vi "generateArrays.vi"(0 "dimension size":i32) -> (8 "errorsWindow1":dbl[](array[numeric]), 10 "pckTotalTrack1":dbl[](array[numeric]), 12 "state1":dbl[](array[numeric]), 14 "errorsWindow2":dbl[](array[numeric]), 15 "pckTotalTrack2":dbl[](array[numeric]), 16 "state2":dbl[](array[numeric]), 17 "errorsWindow3":dbl[](array[numeric]), 18 "pckTotalTrack3":dbl[](array[numeric]), 19 "state3":dbl[](array[numeric]))   [LabVIEW 2010]
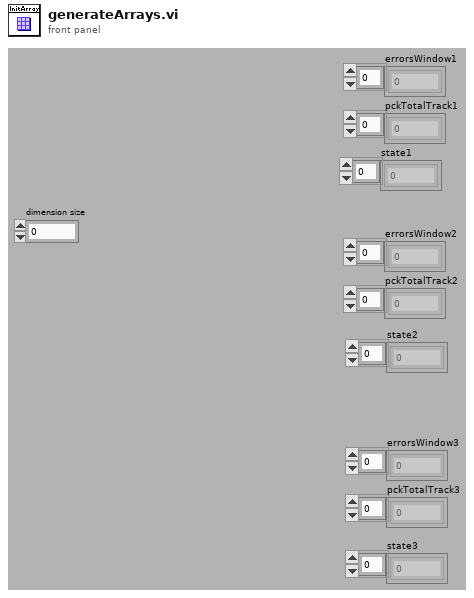
[diagram p1: front panel]
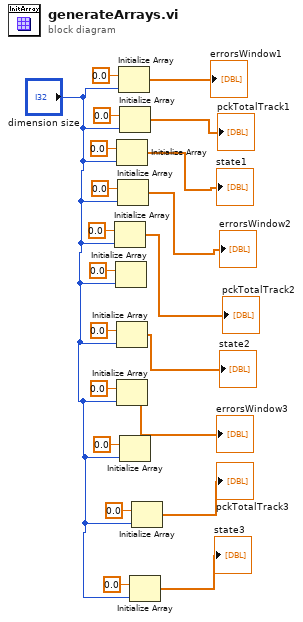
[diagram p0: block diagram]
diagram:
  n1 = Initialize Array(0.0 ("element"), "dimension size") -> (→"pckTotalTrack2":dbl[])
  n2 = Initialize Array(0.0 ("element"), "dimension size") -> ()  [unwired: 1 out]
  n3 = Initialize Array(0.0 ("element"), "dimension size") -> (→"state1":dbl[])
  n4 = Initialize Array(0.0 ("element"), "dimension size") -> (→"state2":dbl[])
  n5 = Initialize Array(0.0 ("element"), "dimension size") -> (→"errorsWindow3":dbl[])
  n6 = Initialize Array(0.0 ("element"), "dimension size") -> (→"errorsWindow2":dbl[])
  n7 = Initialize Array(0.0 ("element"), "dimension size") -> (→"errorsWindow1":dbl[])
  n8 = Initialize Array(0.0 ("element"), "dimension size") -> (→"pckTotalTrack1":dbl[])
  n9 = Initialize Array(0.0 ("element"), "dimension size") -> ()  [unwired: 1 out]
  n10 = Initialize Array(0.0 ("element"), "dimension size") -> (→"state3":dbl[])
  n11 = Initialize Array(0.0 ("element"), "dimension size") -> (→"pckTotalTrack3":dbl[])
